vi "test Loopback_Acyclic_SelectiveTrigger.vi"(8 "error in":errorcluster, 11 "TestCase in":refnum<class "Single Core Acyclic Loopback.lvclass">) -> (0 "error out":errorcluster, 3 "TestCase out":refnum<class "Single Core Acyclic Loopback.lvclass">)   [LabVIEW 2020, in "Single Core Acyclic Loopback.lvclass"]
uses:
  Single Core Acyclic Loopback.lvclass
  C:/Git/niveristand-custom-device-testing-tools/VeriStandTestCase/VeriStandTestCase.lvclass
  <vilib>/numeric/Random Number (Range) I64.vi
  <vilib>/numeric/sub_Random U32.vi
  <vilib>/NI VeriStand/Execution/Workspace/NI VeriStand - Set Multiple Channel Values.vi
  <vilib>/addons/_JKI Toolkits/VI Tester/TestCase.llb/TestCase.lvclass
  <vilib>/NI VeriStand/Execution/Workspace/NI_VS Workspace ExecutionAPI.lvlib
  niveristand-custom-device-testing-tools/VeriStandTestUtilities/VeriStandTestUtilities.lvlib
  C:/Program Files (x86)/National Instruments/LabVIEW 2020/vi.lib/addons/_JKI Toolkits/VI Tester/TestCase.llb/TestCase.lvclass
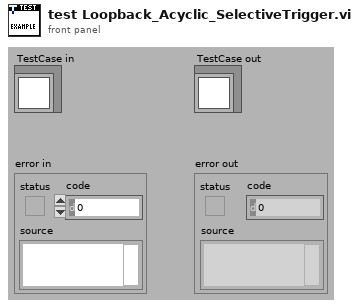
[diagram p1: front panel]
types:
  T1 = typedef "NI_VS Workspace ExecutionAPI.lvlib/WorkspaceAPI.ctl" = refnum<k24>
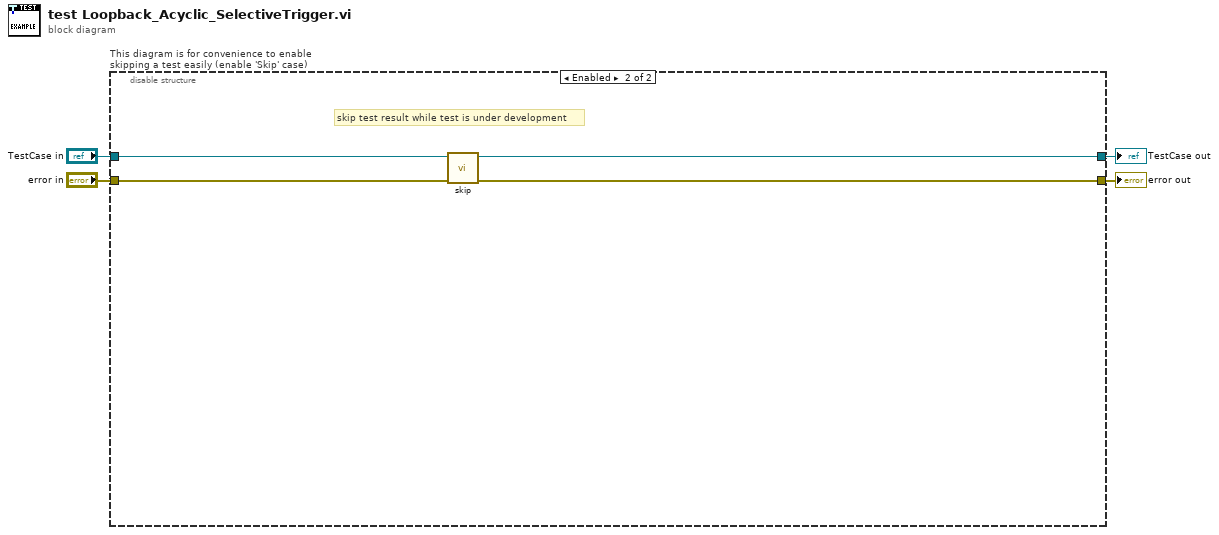
[diagram p0: block diagram]
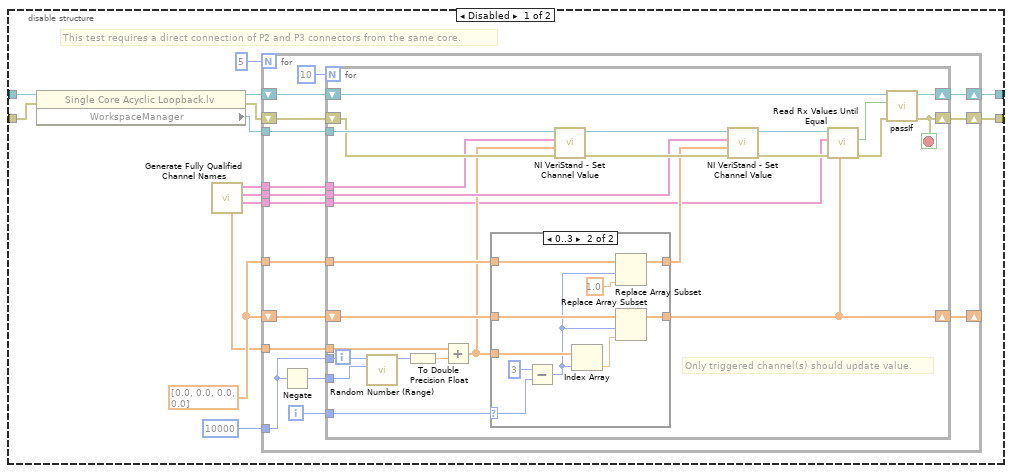
[diagram p2: hidden frame]
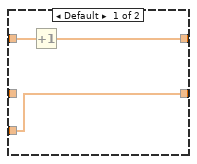
[diagram p3: hidden frame]
diagram:
  n1 = disable-structure "This diagram is for convenience to enable skipping a test easily (enable 'Skip' case)" shown="Enabled" {
    disable-tunnel: "TestCase in" -> [w18 w76]
    disable-tunnel: [w6 w74] -> w1
    disable-tunnel: [w5 w75] -> w3
    disable-tunnel: "error in" -> [w17 w73]
    frame Disabled {
      w11 = dbl[] [0.0, 0.0, 0.0, 0.0] ("Values")
      # "This test requires a direct connection of P2 and P3 connectors from the same core."
      n2 = property class="Single Core Acyclic Loopback.lv"(reference=w18, error in=w17) -> (reference out=w13:refnum<class "Single Core Acyclic Loopback.lvclass">, error out=w14:errorcluster, "WorkspaceManager"=w15:T1)
      n3 = call "Generate Fully Qualified Channel Names.vi"() -> ("Rx channels"=w8:string[], "trigger channels"=w7:string[], "Tx channels"=w10:string[], "channel index"=w9:dbl[])  [unwired: 8 in]
      n4 = for {
        N: 5 -> [_]
        tunnel: w9 -> [w34]
        tunnel: i64 10000 ("upper bound (100)") -> [w33]
        tunnel: w10 -> [w32]
        tunnel: w15 -> [w31]
        tunnel: w8 -> [w29]
        shift-right: [w26] -> w5
        shift-left: w14 -> [w30]
        shift-right: [w27] -> w6
        shift-left: w13 -> [w28]
        tunnel: w7 -> [w24]
        shift-right: [w21] -> _
        shift-left: w11 -> [w23]
        tunnel: w11 -> [w22]
        i -> [w25]
        n5 = Negate(x=w33) -> (-x=w20:i64)
        n6 = for {
          N: 10 -> [_]
          tunnel: w34 -> [w58]
          tunnel: w33 -> [w57]
          tunnel: w20 -> [w56]
          tunnel: w32 -> [w47]
          tunnel: w31 -> [w49]
          tunnel: w29 -> [w35]
          shift-right: [w55] -> w27
          shift-left: w28 -> [w46]
          shift-right: [w54] -> w26
          shift-left: w30 -> [w48]
          tunnel: w25 -> [w44]
          tunnel: w24 -> [w45]
          shift-right: [w36] -> w21
          shift-left: w23 -> [w38]
          tunnel: w22 -> [w39]
          stop <- w54 stop-if-true
          # "Only triggered channel(s) should update value."
          n7 = call-poly <vilib>:"Random Number (Range).vi"("lower bound (-100)"=w56, "upper bound (100)"=w57) -> ("number"=w59:i64)  [unwired: 9 in]
          n8 = To Double Precision Float(number=w59) -> (double precision float=w42:dbl)
          n9 = Add(x=w58, y=w42) -> (x+y=w37:dbl[])
          n10 = case shown="0..3" w44 {
            selector: w44 -> [_ w72]
            tunnel: [w61 w69] -> w43
            tunnel: w39 -> [w62 w68]
            tunnel: w38 -> [_ w67]
            tunnel: w37 -> [w60 w66]
            tunnel: [w60 w64] -> w36
            frame Default {
              n11 = Increment(x=w62) -> (x+1=w61:dbl[])
            }
            frame 0..3 {
              n12 = Subtract(x=3, y=w72) -> (x-y=w63:i32)
              n13 = Index Array(array=w66, index=w63) -> (element=w65:dbl)
              n14 = Replace Array Subset(array=w68, new element=1.0 ("new element/subarray"), index=w63) -> (w69:dbl[])
              n15 = Replace Array Subset(array=w67, new element=w65, index=w63) -> (w64:dbl[])
            }
          }
          n16 = call-poly <vilib>:"NI VeriStand - Set Channel Value.vi"("error in (no error)"=w48, "Values"=w37, "Channels"=w47, "WorkspaceManager in"=w49) -> ("error out"=w50:errorcluster, "WorkspaceManager out"=w53:T1)  [unwired: 6 in]
          n17 = call-poly <vilib>:"NI VeriStand - Set Channel Value.vi"("error in (no error)"=w50, "Values"=w43, "Channels"=w45, "WorkspaceManager in"=w53) -> ("error out"=w51:errorcluster, "WorkspaceManager out"=w52:T1)  [unwired: 6 in]
          n18 = call "Read Rx Values Until Equal.vi"("expected values"=w36, "error in"=w51, "Rx aliases"=w35, "workspace manager in"=w52) -> ("error out"=w40:errorcluster, "values equal expected"=w41:bool)  [unwired: 5 in, 1 out]
          n19 = call-dynamic "passIf.vi"("error in (no error)"=w40, "pass"=w41, "TestCase in"=w46) -> ("error out"=w54:errorcluster, "TestCase out"=w55:refnum<class "Single Core Acyclic Loopback.lvclass">)  [unwired: 7 in]
        }
      }
    }
    frame Enabled {
      # "skip test result while test is under development"
      n20 = call <vilib>:"skip.vi"("error in (no error)"=w73, "TestCase in"=w76) -> ("error out"=w75:errorcluster, "TestCase out"=w74:refnum<class "Single Core Acyclic Loopback.lvclass">)  [unwired: 8 in]
    }
  }
  "error out" <- w3
  "TestCase out" <- w1
